vi "Fetch Waveform Measurement [WM].vi"(8 "error in (no error)":errorcluster, 9 "measurement function (Rise Time)":i32(ring) items=["Rise Time"=0, "Fall Time"=1, "Frequency"=2, "Period"=3, "Voltage RMS"=4, "Voltage RMS (cycle)"=16, "Voltage Min"=7, "Voltage Max"=6, "Voltage Vpp"=5, "Voltage Low"=9, "Voltage High"=8, "Voltage Average"=10, "Voltage Average (cycle)"=17, "Width Negative"=11, "Width Positive"=12, "Duty Cycle Negative"=13, "Duty Cycle Positive"=14, "Amplitude"=15, "Overshoot"=18, "Preshoot"=19], 10 "channel name (\"CHANNEL1\")":string="CHANNEL1", 11 "CS++Scope":refnum<class "CS++Scope.lvclass">) -> (0 "error out":errorcluster, 2 "measurement":dbl format="%^.2e", 3 "CS++Scope out":refnum<class "CS++Scope.lvclass">)   [LabVIEW 2016, in "CS++Scope.lvlib" / "CS++Scope.lvclass"]
doc: "This VI fetches a waveform measurement from the channel you specify. If the channel is not enabled for the acquisition, this VI returns IVISCOPE_ERROR_CHANNEL_NOT_ENABLED (0xBFFA2001) error.\nThe waveform on which the oscilloscope calculates the waveform measurement is from an acquisition that you previously initiated.\nUse the IviScope Initiate Acquisition VI to start an acquisition on the channels that you enable with the IviScope Configure Channel VI. The oscilloscope acquires waveforms for the enabled channels concurrently. You use the IviScope Acquisition Status VI to determine when the acquisition is complete. You call this VI separately for each waveform measurement you want to obtain on a specific channel.\n\nYou can call the IviScope Read Waveform Measurement [WM] VI instead of the IviScope Initiate Acquisition VI. The IviScope Read Waveform Measurement [WM] VI starts an acquisition on all enabled channels. It then waits for the acquisition to complete, obtains a waveform measurement on the channel you specify, and returns the measurement value. You call this VI separately for any other waveform measurement that you want to obtain on a specific channel.\n\nNotes:\n(1) You must configure the appropriate reference levels before you call this VI. You configure the low, mid, and high references either by calling the IviScope Configure Reference Levels [WM] VI or by setting the following properties.\nIviScope>>Waveform Measurement [WM]>> Measurement High Reference [WM]\nIviScope>>Waveform Measurement [WM]>> Measurement Low Reference [WM]\nIviScope>>Waveform Measurement [WM]>> Measurement Mid Reference [WM]\n\n(2) This VI does not check the instrument status. Typically, you call this VI only in a sequence of calls to other low-level driver VIs. The sequence performs one operation. You use the low-level VIs to optimize one or more aspects of interaction with the instrument. If you want to check the instrument status, call the IviScope Error-Query VI at the conclusion of the sequence.\n\n(3) The class driver returns a simulated measurement when this VI is called and the IviScope>>Inherent IVI Settings>>User Options>>Simulate property is set to TRUE and the IviScope>>Inherent IVI Settings>>User Options>>Use Specific Simulation property is set to FALSE. For information on how to configure a simulated measurement, refer to the online help manual.\n\n(4) This VI is part of the IviScopeWaveformMeasurement [WM] extension group."
uses:
  CS++Scope.lvclass
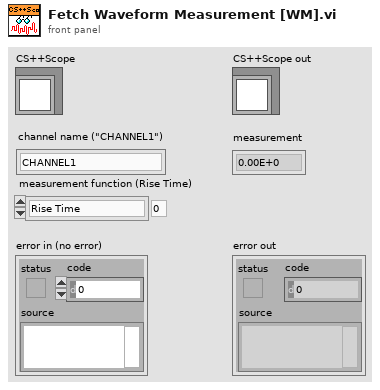
[diagram p1: front panel]
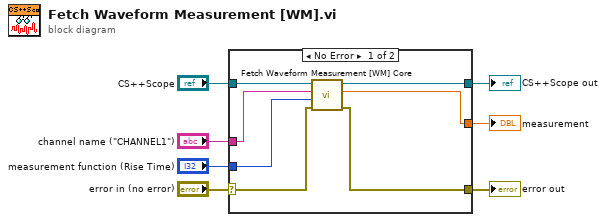
[diagram p0: block diagram]
diagram:
  n1 = case shown="No Error" "error in (no error)" {
    selector: "error in (no error)" -> [w12 w16]
    tunnel: [w11 w16] -> w6
    tunnel: [w13 w15] -> w3
    tunnel: "CS++Scope" -> [w14 w15]
    tunnel: "channel name (\"CHANNEL1\")" -> [w10 _]
    tunnel: "measurement function (Rise Time)" -> [w9 _]
    tunnel: [w8 _] -> w1
    frame No Error {
      n2 = call-dynamic "Fetch Waveform Measurement [WM] Core.vi"("error in (no error)"=w12, "measurement function (Rise Time)"=w9, "channel name (\"CHANNEL1\")"=w10, "CS++Scope"=w14) -> ("error out"=w11:errorcluster, "measurement"=w8:dbl, "CS++Scope out"=w13:refnum<class "CS++Scope.lvclass">)  [unwired: 5 in]
    }
    frame Error {
    }
  }
  "error out" <- w6
  "measurement" <- w1
  "CS++Scope out" <- w3
